vi "Next command.vi"(8 "error in (no error)":errorcluster, 11 "Channel in":refnum<class "Channel.lvclass">) -> (0 "error out":errorcluster, 3 "Channel out":refnum<class "Channel.lvclass">)   [LabVIEW 2018, in "Channel.lvclass"]
uses:
  Channel.lvclass
  Channel.lvclass/Channel.ctl
  State Machine/State Machine.lvclass/State Machine.ctl
  File interpreter/File interpreter.lvclass
  RxTx/RxTx.lvclass
  Interface/Interface.lvclass
  State Machine/State Machine.lvclass
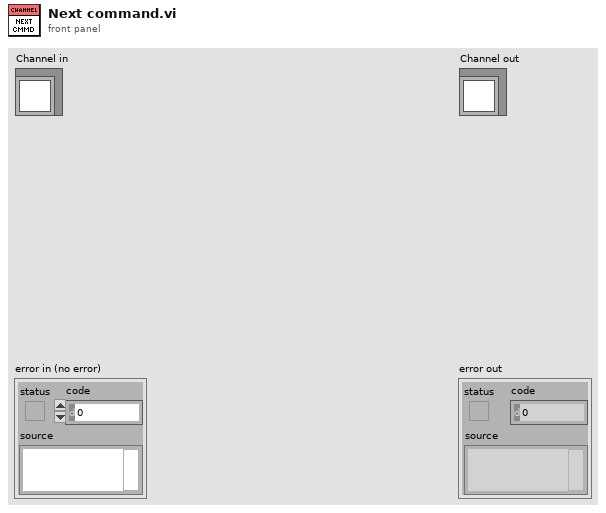
[diagram p1: front panel]
types:
  T1 = typedef "Shutter_mode typedef.ctl" = enum16{"Auto", "Open", "Close", "N/A (3)", "Open FVB Series", "Open Any Series"}
  T2 = typedef "ReadMode_mode typedef.ctl" = enum16{"Full Vertical Binning", "Multi-Track", "Random-Track", "Single-Track", "Image"}
  T3 = typedef "AcquisitionMode_mode typedef.ctl" = enum16{"Reserved (0)", "Single Scan", "Accumulate", "Kinetics", "Fast Kinetics", "Run Till Abort", "Reserved (6)", "Reserved (7)", "Reserved (8)", "Time Delayed Integration"}
  T4 = cluster{"EXPTIME":sgl, "PREAMP":enum16{"Gain 1", "Gain 2"}, "READOUT_RATE":enum16{"30 MHz", "20 MHz", "10 MHz", "1 MHz"}, "EM_GAIN":u16, "VBIN":u16, "INITIAL_LINE":u16, "INITIAL_COLUMN":u16, "FINAL_LINE":u16, "FINAL_COLUMN":u16, "#FRAMES":u32, "#CUBES":u32, "TRIGGER_MODE":enum16{"Internal", "External", "N/A", "N/A_1", "N/A_2", "N/A_3", "External Start"}, "HBIN":u16, "SHUTTER_TTL":enum16{"TTL Low", "TTL High"}, "SHUTTER_MODE":T1, "SHUTTER_OPENING_TIME":u16, "SHUTTER_CLOSING_TIME":u16, "VERTICAL_SHIFT_SPEED":u16, "READ_MODE":T2, "FRAME_TRANSFER":bool, "VERTICAL_CLOCK_VOLTAGE":enum16{"0", "+1", "+2", "+3", "+4"}, "ACQUISITION_MODE":T3, "AD_CHANNEL":u16, "EM_MODE":enum16{"Electron Multiplying", "Conventional"}}
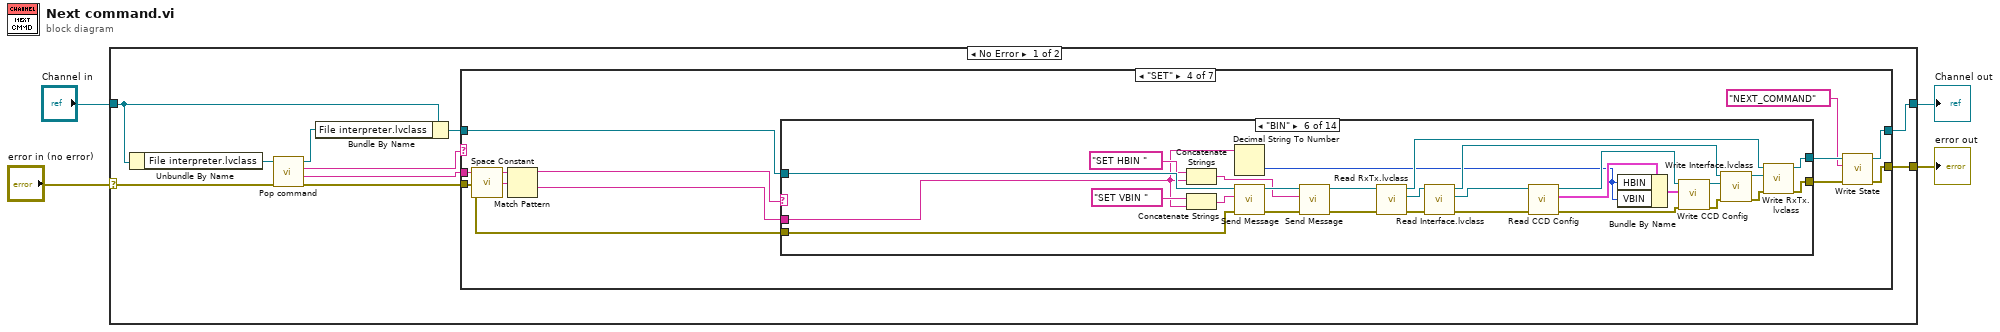
[diagram p0: block diagram]
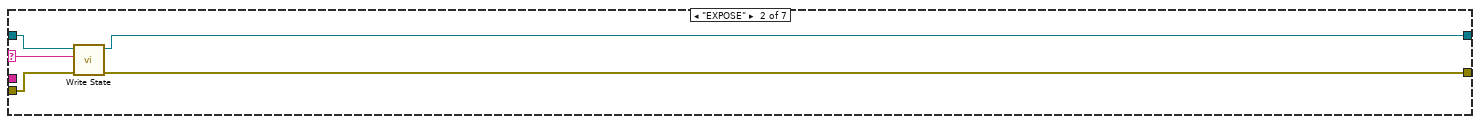
[diagram p3: hidden frame]
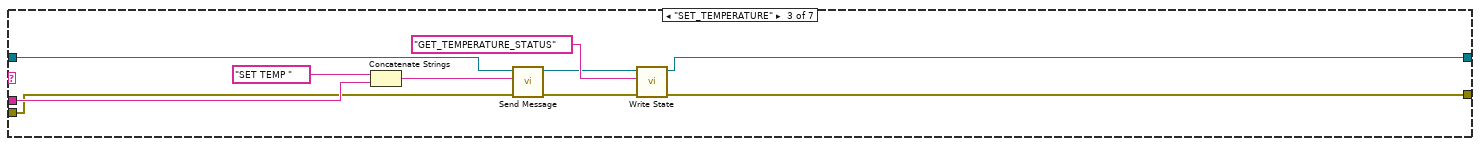
[diagram p4: hidden frame]
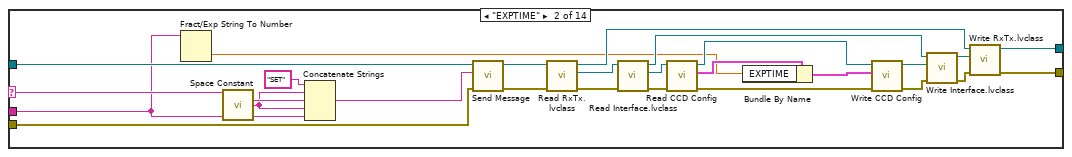
[diagram p6: hidden frame]
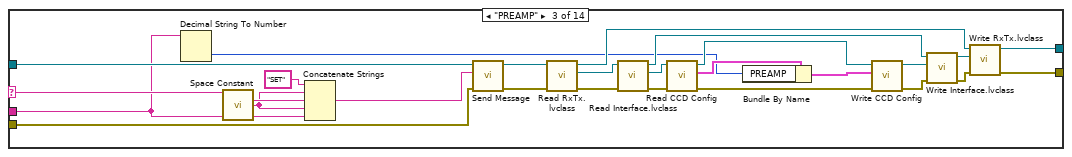
[diagram p7: hidden frame]
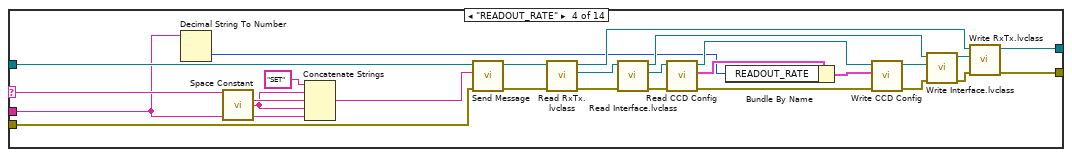
[diagram p8: hidden frame]
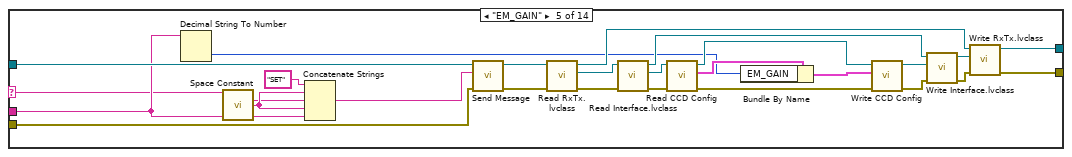
[diagram p9: hidden frame]
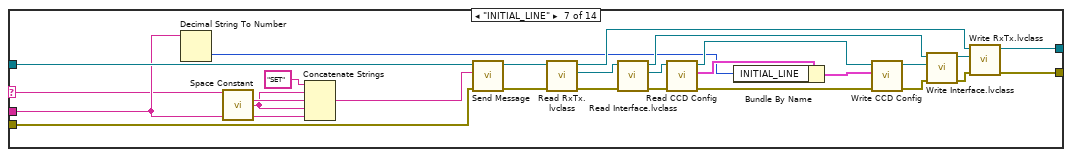
[diagram p10: hidden frame]
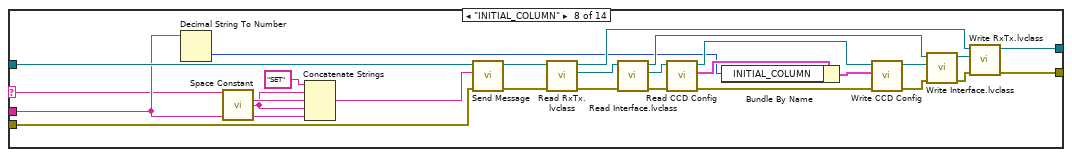
[diagram p11: hidden frame]
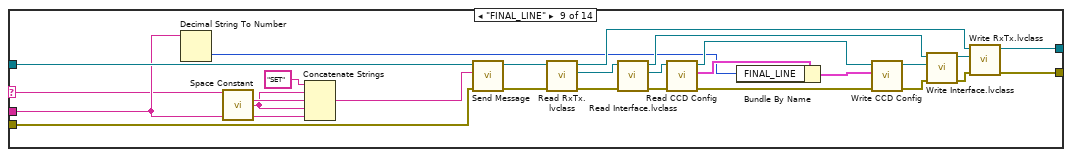
[diagram p12: hidden frame]
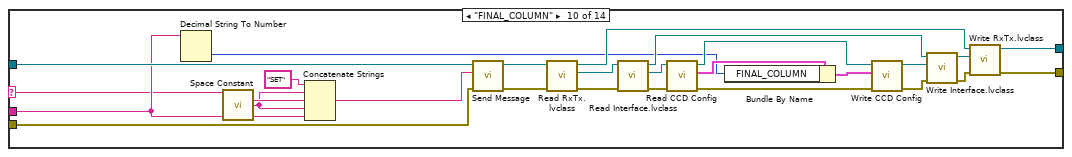
[diagram p13: hidden frame]
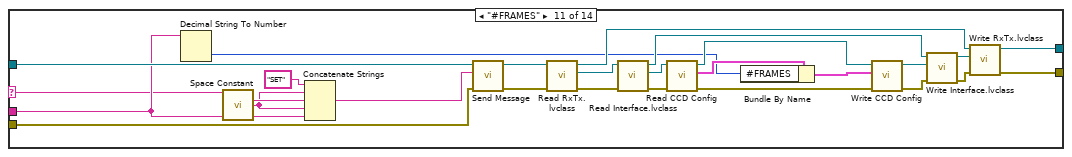
[diagram p14: hidden frame]
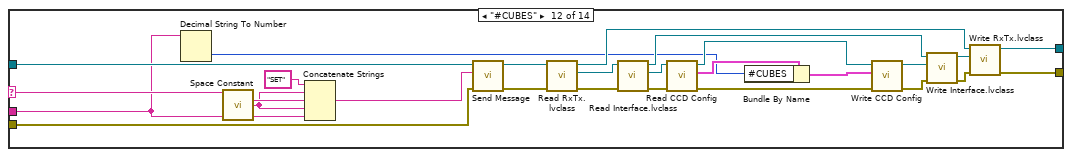
[diagram p15: hidden frame]
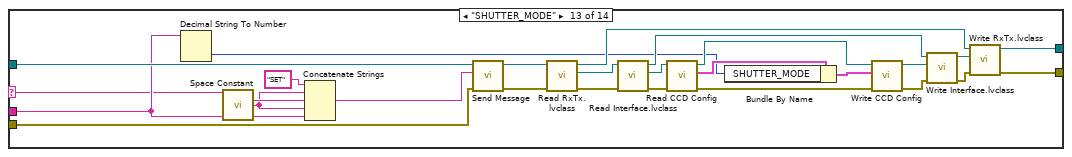
[diagram p16: hidden frame]
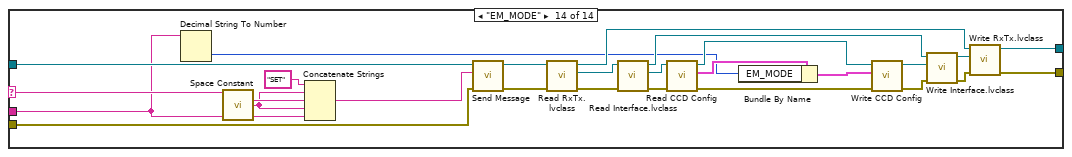
[diagram p17: hidden frame]
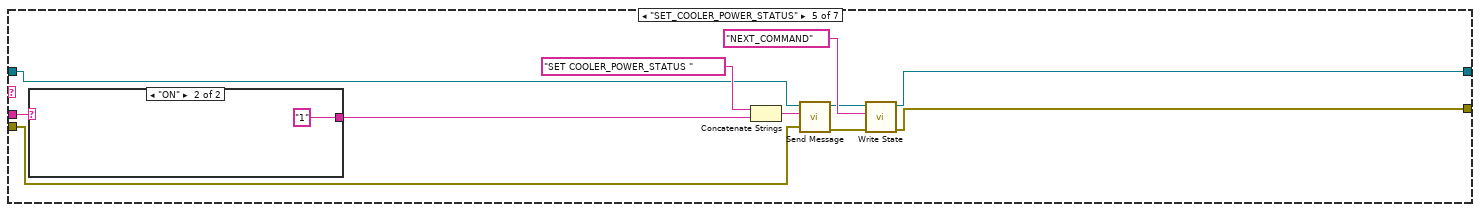
[diagram p18: hidden frame]
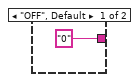
[diagram p19: hidden frame]
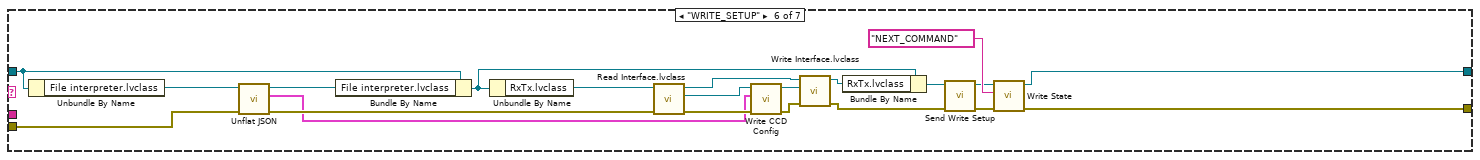
[diagram p20: hidden frame]
diagram:
  n1 = case shown="No Error" "error in (no error)" {
    selector: "error in (no error)" -> [w14 w433]
    tunnel: [w8 w433] -> w3
    tunnel: [w9 w432] -> w1
    tunnel: "Channel in" -> [w11 w432]
    frame No Error {
      n2 = Unbundle By Name(w11) -> ("File interpreter.lvclass"=w13:refnum<class "File interpreter.lvclass">)
      n3 = call "Pop command.vi"("error in (no error)"=w14, "File interpreter in"=w13) -> ("error out"=w10:errorcluster, "Value"=w5:string, "command"=w6:string, "File interpreter out"=w12:refnum<class "File interpreter.lvclass">)  [unwired: 6 in]
      n4 = Bundle By Name(cluster=w11, "File interpreter.lvclass"=w12) -> (w7:refnum<class "Channel.lvclass">)
      n5 = case shown="\"SET\"" w6 {
        selector: w6 -> [_ w17 _ _ _ _ _]
        tunnel: w7 -> [w16 w21 w25 w42 w390 w415 w431]
        tunnel: w10 -> [w15 w20 w22 w41 w387 w418 w428]
        tunnel: [w16 w19 w31 w35 w395 w403 w422] -> w9
        tunnel: [w15 w18 w30 w34 w394 w404 w421] -> w8
        tunnel: w5 -> [_ _ w26 w40 w386 _ w427]
        frame "False", Default {
        }
        frame "EXPOSE" {
          n6 = call "Write State.vi"("error in (no error)"=w20, "State"=w17, "Channel in"=w21) -> ("error out"=w18:errorcluster, "Channel out"=w19:refnum<class "Channel.lvclass">)  [unwired: 7 in]
        }
        frame "SET_TEMPERATURE" {
          n7 = Concatenate Strings("SET TEMP ", w26) -> (w28:string)
          n8 = call "Send Message.vi"("error in (no error)"=w22, "message"=w28, "Channel in"=w25) -> ("error out"=w23:errorcluster, "Channel out"=w24:refnum<class "Channel.lvclass">)  [unwired: 7 in]
          n9 = call "Write State.vi"("error in (no error)"=w23, "State"="GET_TEMPERATURE_STATUS", "Channel in"=w24) -> ("error out"=w30:errorcluster, "Channel out"=w31:refnum<class "Channel.lvclass">)  [unwired: 7 in]
        }
        frame "SET" {
          n10 = call <vilib>:"Space Constant.vi"() -> ("String"=w39:string)
          n11 = Match Pattern(string=w40, regular expression=w39) -> (before substring=w38:string, after substring=w37:string)  [unwired: 1 in, 2 out]
          n12 = case shown="\"BIN\"" w38 {
            selector: w38 -> [_ w48 w74 w100 w123 _ w179 w205 w231 w257 w283 w310 w335 w362]
            tunnel: [w44 w58 w84 w110 w136 w164 w190 w216 w242 w268 w294 w320 w346 w372] -> w36
            tunnel: [w43 w57 w83 w109 w135 w163 w189 w215 w241 w267 w293 w319 w345 w371] -> w33
            tunnel: w42 -> [w44 w51 w77 w103 w129 w160 w184 w210 w236 w262 w288 w314 w340 w366]
            tunnel: w41 -> [w43 w50 w76 w102 w128 w159 w183 w209 w235 w261 w287 w313 w339 w365]
            tunnel: w37 -> [_ w47 w73 w99 w126 w149 w180 w206 w232 w258 w284 w307 w336 w359]
            frame "False", Default {
            }
            frame "EXPTIME" {
              n13 = Fract/Exp String To Number(string=w47) -> (number=w54:dbl)  [unwired: 3 in, 1 out]
              n14 = call <vilib>:"Space Constant.vi"() -> ("String"=w46:string)
              n15 = Concatenate Strings("SET" ("string"), w46, w48, w46, w47) -> (w49:string)
              n16 = call "Send Message.vi"("error in (no error)"=w50, "message"=w49, "Channel in"=w51) -> ("error out"=w52:errorcluster, "Channel out"=w53:refnum<class "Channel.lvclass">)  [unwired: 7 in]
              n17 = call "Read RxTx.lvclass.vi"("error in (no error)"=w52, "Channel in"=w53) -> ("error out"=w60:errorcluster, "RxTx.lvclass"=w70:refnum<class "RxTx.lvclass">, "Channel out"=w65:refnum<class "Channel.lvclass">)  [unwired: 7 in]
              n18 = call "Read Interface.lvclass.vi"("error in (no error)"=w60, "RxTx in"=w70) -> ("error out"=w61:errorcluster, "Interface.lvclass"=w69:refnum<class "Interface.lvclass">, "RxTx out"=w64:refnum<class "RxTx.lvclass">)  [unwired: 7 in]
              n19 = call "Read CCD Config.vi"("error in (no error)"=w61, "Interface in"=w69) -> ("error out"=w59:errorcluster, "CCD Config"=w56:T4, "Interface out"=w68:refnum<class "Interface.lvclass">)  [unwired: 7 in]
              n20 = Bundle By Name(cluster=w56, "EXPTIME"=w54) -> (w55:T4)
              n21 = call "Write CCD Config.vi"("error in (no error)"=w59, "CCD Config"=w55, "Interface in"=w68) -> ("error out"=w62:errorcluster, "Interface out"=w67:refnum<class "Interface.lvclass">)  [unwired: 7 in]
              n22 = call "Write Interface.lvclass.vi"("error in (no error)"=w62, "Interface.lvclass"=w67, "RxTx in"=w64) -> ("error out"=w63:errorcluster, "RxTx out"=w66:refnum<class "RxTx.lvclass">)  [unwired: 7 in]
              n23 = call "Write RxTx.lvclass.vi"("error in (no error)"=w63, "RxTx.lvclass"=w66, "Channel in"=w65) -> ("error out"=w57:errorcluster, "Channel out"=w58:refnum<class "Channel.lvclass">)  [unwired: 7 in]
            }
            frame "PREAMP" {
              n24 = Decimal String To Number(string=w73) -> (number=w80:i32)  [unwired: 2 in, 1 out]
              n25 = call <vilib>:"Space Constant.vi"() -> ("String"=w72:string)
              n26 = Concatenate Strings("SET" ("string"), w72, w74, w72, w73) -> (w75:string)
              n27 = call "Send Message.vi"("error in (no error)"=w76, "message"=w75, "Channel in"=w77) -> ("error out"=w78:errorcluster, "Channel out"=w79:refnum<class "Channel.lvclass">)  [unwired: 7 in]
              n28 = call "Read RxTx.lvclass.vi"("error in (no error)"=w78, "Channel in"=w79) -> ("error out"=w86:errorcluster, "RxTx.lvclass"=w96:refnum<class "RxTx.lvclass">, "Channel out"=w91:refnum<class "Channel.lvclass">)  [unwired: 7 in]
              n29 = call "Read Interface.lvclass.vi"("error in (no error)"=w86, "RxTx in"=w96) -> ("error out"=w87:errorcluster, "Interface.lvclass"=w95:refnum<class "Interface.lvclass">, "RxTx out"=w90:refnum<class "RxTx.lvclass">)  [unwired: 7 in]
              n30 = call "Read CCD Config.vi"("error in (no error)"=w87, "Interface in"=w95) -> ("error out"=w85:errorcluster, "CCD Config"=w82:T4, "Interface out"=w94:refnum<class "Interface.lvclass">)  [unwired: 7 in]
              n31 = Bundle By Name(cluster=w82, "PREAMP"=w80) -> (w81:T4)
              n32 = call "Write CCD Config.vi"("error in (no error)"=w85, "CCD Config"=w81, "Interface in"=w94) -> ("error out"=w88:errorcluster, "Interface out"=w93:refnum<class "Interface.lvclass">)  [unwired: 7 in]
              n33 = call "Write Interface.lvclass.vi"("error in (no error)"=w88, "Interface.lvclass"=w93, "RxTx in"=w90) -> ("error out"=w89:errorcluster, "RxTx out"=w92:refnum<class "RxTx.lvclass">)  [unwired: 7 in]
              n34 = call "Write RxTx.lvclass.vi"("error in (no error)"=w89, "RxTx.lvclass"=w92, "Channel in"=w91) -> ("error out"=w83:errorcluster, "Channel out"=w84:refnum<class "Channel.lvclass">)  [unwired: 7 in]
            }
            frame "READOUT_RATE" {
              n35 = Decimal String To Number(string=w99) -> (number=w106:i32)  [unwired: 2 in, 1 out]
              n36 = call <vilib>:"Space Constant.vi"() -> ("String"=w98:string)
              n37 = Concatenate Strings("SET" ("string"), w98, w100, w98, w99) -> (w101:string)
              n38 = call "Send Message.vi"("error in (no error)"=w102, "message"=w101, "Channel in"=w103) -> ("error out"=w104:errorcluster, "Channel out"=w105:refnum<class "Channel.lvclass">)  [unwired: 7 in]
              n39 = call "Read RxTx.lvclass.vi"("error in (no error)"=w104, "Channel in"=w105) -> ("error out"=w112:errorcluster, "RxTx.lvclass"=w122:refnum<class "RxTx.lvclass">, "Channel out"=w117:refnum<class "Channel.lvclass">)  [unwired: 7 in]
              n40 = call "Read Interface.lvclass.vi"("error in (no error)"=w112, "RxTx in"=w122) -> ("error out"=w113:errorcluster, "Interface.lvclass"=w121:refnum<class "Interface.lvclass">, "RxTx out"=w116:refnum<class "RxTx.lvclass">)  [unwired: 7 in]
              n41 = call "Read CCD Config.vi"("error in (no error)"=w113, "Interface in"=w121) -> ("error out"=w111:errorcluster, "CCD Config"=w108:T4, "Interface out"=w120:refnum<class "Interface.lvclass">)  [unwired: 7 in]
              n42 = Bundle By Name(cluster=w108, "READOUT_RATE"=w106) -> (w107:T4)
              n43 = call "Write CCD Config.vi"("error in (no error)"=w111, "CCD Config"=w107, "Interface in"=w120) -> ("error out"=w114:errorcluster, "Interface out"=w119:refnum<class "Interface.lvclass">)  [unwired: 7 in]
              n44 = call "Write Interface.lvclass.vi"("error in (no error)"=w114, "Interface.lvclass"=w119, "RxTx in"=w116) -> ("error out"=w115:errorcluster, "RxTx out"=w118:refnum<class "RxTx.lvclass">)  [unwired: 7 in]
              n45 = call "Write RxTx.lvclass.vi"("error in (no error)"=w115, "RxTx.lvclass"=w118, "Channel in"=w117) -> ("error out"=w109:errorcluster, "Channel out"=w110:refnum<class "Channel.lvclass">)  [unwired: 7 in]
            }
            frame "EM_GAIN" {
              n46 = Decimal String To Number(string=w126) -> (number=w132:i32)  [unwired: 2 in, 1 out]
              n47 = call <vilib>:"Space Constant.vi"() -> ("String"=w124:string)
              n48 = Concatenate Strings("SET" ("string"), w124, w123, w124, w126) -> (w127:string)
              n49 = call "Send Message.vi"("error in (no error)"=w128, "message"=w127, "Channel in"=w129) -> ("error out"=w130:errorcluster, "Channel out"=w131:refnum<class "Channel.lvclass">)  [unwired: 7 in]
              n50 = call "Read RxTx.lvclass.vi"("error in (no error)"=w130, "Channel in"=w131) -> ("error out"=w138:errorcluster, "RxTx.lvclass"=w148:refnum<class "RxTx.lvclass">, "Channel out"=w143:refnum<class "Channel.lvclass">)  [unwired: 7 in]
              n51 = call "Read Interface.lvclass.vi"("error in (no error)"=w138, "RxTx in"=w148) -> ("error out"=w139:errorcluster, "Interface.lvclass"=w147:refnum<class "Interface.lvclass">, "RxTx out"=w142:refnum<class "RxTx.lvclass">)  [unwired: 7 in]
              n52 = call "Read CCD Config.vi"("error in (no error)"=w139, "Interface in"=w147) -> ("error out"=w137:errorcluster, "CCD Config"=w134:T4, "Interface out"=w146:refnum<class "Interface.lvclass">)  [unwired: 7 in]
              n53 = Bundle By Name(cluster=w134, "EM_GAIN"=w132) -> (w133:T4)
              n54 = call "Write CCD Config.vi"("error in (no error)"=w137, "CCD Config"=w133, "Interface in"=w146) -> ("error out"=w140:errorcluster, "Interface out"=w145:refnum<class "Interface.lvclass">)  [unwired: 7 in]
              n55 = call "Write Interface.lvclass.vi"("error in (no error)"=w140, "Interface.lvclass"=w145, "RxTx in"=w142) -> ("error out"=w141:errorcluster, "RxTx out"=w144:refnum<class "RxTx.lvclass">)  [unwired: 7 in]
              n56 = call "Write RxTx.lvclass.vi"("error in (no error)"=w141, "RxTx.lvclass"=w144, "Channel in"=w143) -> ("error out"=w135:errorcluster, "Channel out"=w136:refnum<class "Channel.lvclass">)  [unwired: 7 in]
            }
            frame "BIN" {
              n57 = Concatenate Strings("SET HBIN " ("string"), w149) -> (w150:string)
              n58 = Concatenate Strings("SET VBIN " ("string"), w149) -> (w158:string)
              n59 = Decimal String To Number(string=w149) -> (number=w157:i32)  [unwired: 2 in, 1 out]
              n60 = call "Send Message.vi"("error in (no error)"=w159, "message"=w158, "Channel in"=w160) -> ("error out"=w152:errorcluster, "Channel out"=w155:refnum<class "Channel.lvclass">)  [unwired: 7 in]
              n61 = call "Send Message.vi"("error in (no error)"=w152, "message"=w150, "Channel in"=w155) -> ("error out"=w153:errorcluster, "Channel out"=w154:refnum<class "Channel.lvclass">)  [unwired: 7 in]
              n62 = call "Read RxTx.lvclass.vi"("error in (no error)"=w153, "Channel in"=w154) -> ("error out"=w166:errorcluster, "RxTx.lvclass"=w176:refnum<class "RxTx.lvclass">, "Channel out"=w171:refnum<class "Channel.lvclass">)  [unwired: 7 in]
              n63 = call "Read Interface.lvclass.vi"("error in (no error)"=w166, "RxTx in"=w176) -> ("error out"=w167:errorcluster, "Interface.lvclass"=w175:refnum<class "Interface.lvclass">, "RxTx out"=w170:refnum<class "RxTx.lvclass">)  [unwired: 7 in]
              n64 = call "Read CCD Config.vi"("error in (no error)"=w167, "Interface in"=w175) -> ("error out"=w165:errorcluster, "CCD Config"=w162:T4, "Interface out"=w174:refnum<class "Interface.lvclass">)  [unwired: 7 in]
              n65 = Bundle By Name(cluster=w162, "HBIN"=w157, "VBIN"=w157) -> (w161:T4)
              n66 = call "Write CCD Config.vi"("error in (no error)"=w165, "CCD Config"=w161, "Interface in"=w174) -> ("error out"=w168:errorcluster, "Interface out"=w173:refnum<class "Interface.lvclass">)  [unwired: 7 in]
              n67 = call "Write Interface.lvclass.vi"("error in (no error)"=w168, "Interface.lvclass"=w173, "RxTx in"=w170) -> ("error out"=w169:errorcluster, "RxTx out"=w172:refnum<class "RxTx.lvclass">)  [unwired: 7 in]
              n68 = call "Write RxTx.lvclass.vi"("error in (no error)"=w169, "RxTx.lvclass"=w172, "Channel in"=w171) -> ("error out"=w163:errorcluster, "Channel out"=w164:refnum<class "Channel.lvclass">)  [unwired: 7 in]
            }
            frame "INITIAL_LINE" {
              n69 = Decimal String To Number(string=w180) -> (number=w181:i32)  [unwired: 2 in, 1 out]
              n70 = call <vilib>:"Space Constant.vi"() -> ("String"=w178:string)
              n71 = Concatenate Strings("SET" ("string"), w178, w179, w178, w180) -> (w182:string)
              n72 = call "Send Message.vi"("error in (no error)"=w183, "message"=w182, "Channel in"=w184) -> ("error out"=w185:errorcluster, "Channel out"=w186:refnum<class "Channel.lvclass">)  [unwired: 7 in]
              n73 = call "Read RxTx.lvclass.vi"("error in (no error)"=w185, "Channel in"=w186) -> ("error out"=w192:errorcluster, "RxTx.lvclass"=w202:refnum<class "RxTx.lvclass">, "Channel out"=w197:refnum<class "Channel.lvclass">)  [unwired: 7 in]
              n74 = call "Read Interface.lvclass.vi"("error in (no error)"=w192, "RxTx in"=w202) -> ("error out"=w193:errorcluster, "Interface.lvclass"=w201:refnum<class "Interface.lvclass">, "RxTx out"=w196:refnum<class "RxTx.lvclass">)  [unwired: 7 in]
              n75 = call "Read CCD Config.vi"("error in (no error)"=w193, "Interface in"=w201) -> ("error out"=w191:errorcluster, "CCD Config"=w188:T4, "Interface out"=w200:refnum<class "Interface.lvclass">)  [unwired: 7 in]
              n76 = Bundle By Name(cluster=w188, "INITIAL_LINE"=w181) -> (w187:T4)
              n77 = call "Write CCD Config.vi"("error in (no error)"=w191, "CCD Config"=w187, "Interface in"=w200) -> ("error out"=w194:errorcluster, "Interface out"=w199:refnum<class "Interface.lvclass">)  [unwired: 7 in]
              n78 = call "Write Interface.lvclass.vi"("error in (no error)"=w194, "Interface.lvclass"=w199, "RxTx in"=w196) -> ("error out"=w195:errorcluster, "RxTx out"=w198:refnum<class "RxTx.lvclass">)  [unwired: 7 in]
              n79 = call "Write RxTx.lvclass.vi"("error in (no error)"=w195, "RxTx.lvclass"=w198, "Channel in"=w197) -> ("error out"=w189:errorcluster, "Channel out"=w190:refnum<class "Channel.lvclass">)  [unwired: 7 in]
            }
            frame "INITIAL_COLUMN" {
              n80 = Decimal String To Number(string=w206) -> (number=w207:i32)  [unwired: 2 in, 1 out]
              n81 = call <vilib>:"Space Constant.vi"() -> ("String"=w204:string)
              n82 = Concatenate Strings("SET" ("string"), w204, w205, w204, w206) -> (w208:string)
              n83 = call "Send Message.vi"("error in (no error)"=w209, "message"=w208, "Channel in"=w210) -> ("error out"=w211:errorcluster, "Channel out"=w212:refnum<class "Channel.lvclass">)  [unwired: 7 in]
              n84 = call "Read RxTx.lvclass.vi"("error in (no error)"=w211, "Channel in"=w212) -> ("error out"=w218:errorcluster, "RxTx.lvclass"=w228:refnum<class "RxTx.lvclass">, "Channel out"=w223:refnum<class "Channel.lvclass">)  [unwired: 7 in]
              n85 = call "Read Interface.lvclass.vi"("error in (no error)"=w218, "RxTx in"=w228) -> ("error out"=w219:errorcluster, "Interface.lvclass"=w227:refnum<class "Interface.lvclass">, "RxTx out"=w222:refnum<class "RxTx.lvclass">)  [unwired: 7 in]
              n86 = call "Read CCD Config.vi"("error in (no error)"=w219, "Interface in"=w227) -> ("error out"=w217:errorcluster, "CCD Config"=w214:T4, "Interface out"=w226:refnum<class "Interface.lvclass">)  [unwired: 7 in]
              n87 = Bundle By Name(cluster=w214, "INITIAL_COLUMN"=w207) -> (w213:T4)
              n88 = call "Write CCD Config.vi"("error in (no error)"=w217, "CCD Config"=w213, "Interface in"=w226) -> ("error out"=w220:errorcluster, "Interface out"=w225:refnum<class "Interface.lvclass">)  [unwired: 7 in]
              n89 = call "Write Interface.lvclass.vi"("error in (no error)"=w220, "Interface.lvclass"=w225, "RxTx in"=w222) -> ("error out"=w221:errorcluster, "RxTx out"=w224:refnum<class "RxTx.lvclass">)  [unwired: 7 in]
              n90 = call "Write RxTx.lvclass.vi"("error in (no error)"=w221, "RxTx.lvclass"=w224, "Channel in"=w223) -> ("error out"=w215:errorcluster, "Channel out"=w216:refnum<class "Channel.lvclass">)  [unwired: 7 in]
            }
            frame "FINAL_LINE" {
              n91 = Decimal String To Number(string=w232) -> (number=w233:i32)  [unwired: 2 in, 1 out]
              n92 = call <vilib>:"Space Constant.vi"() -> ("String"=w230:string)
              n93 = Concatenate Strings("SET" ("string"), w230, w231, w230, w232) -> (w234:string)
              n94 = call "Send Message.vi"("error in (no error)"=w235, "message"=w234, "Channel in"=w236) -> ("error out"=w237:errorcluster, "Channel out"=w238:refnum<class "Channel.lvclass">)  [unwired: 7 in]
              n95 = call "Read RxTx.lvclass.vi"("error in (no error)"=w237, "Channel in"=w238) -> ("error out"=w244:errorcluster, "RxTx.lvclass"=w254:refnum<class "RxTx.lvclass">, "Channel out"=w249:refnum<class "Channel.lvclass">)  [unwired: 7 in]
              n96 = call "Read Interface.lvclass.vi"("error in (no error)"=w244, "RxTx in"=w254) -> ("error out"=w245:errorcluster, "Interface.lvclass"=w253:refnum<class "Interface.lvclass">, "RxTx out"=w248:refnum<class "RxTx.lvclass">)  [unwired: 7 in]
              n97 = call "Read CCD Config.vi"("error in (no error)"=w245, "Interface in"=w253) -> ("error out"=w243:errorcluster, "CCD Config"=w240:T4, "Interface out"=w252:refnum<class "Interface.lvclass">)  [unwired: 7 in]
              n98 = Bundle By Name(cluster=w240, "FINAL_LINE"=w233) -> (w239:T4)
              n99 = call "Write CCD Config.vi"("error in (no error)"=w243, "CCD Config"=w239, "Interface in"=w252) -> ("error out"=w246:errorcluster, "Interface out"=w251:refnum<class "Interface.lvclass">)  [unwired: 7 in]
              n100 = call "Write Interface.lvclass.vi"("error in (no error)"=w246, "Interface.lvclass"=w251, "RxTx in"=w248) -> ("error out"=w247:errorcluster, "RxTx out"=w250:refnum<class "RxTx.lvclass">)  [unwired: 7 in]
              n101 = call "Write RxTx.lvclass.vi"("error in (no error)"=w247, "RxTx.lvclass"=w250, "Channel in"=w249) -> ("error out"=w241:errorcluster, "Channel out"=w242:refnum<class "Channel.lvclass">)  [unwired: 7 in]
            }
            frame "FINAL_COLUMN" {
              n102 = Decimal String To Number(string=w258) -> (number=w259:i32)  [unwired: 2 in, 1 out]
              n103 = call <vilib>:"Space Constant.vi"() -> ("String"=w256:string)
              n104 = Concatenate Strings("SET" ("string"), w256, w257, w256, w258) -> (w260:string)
              n105 = call "Send Message.vi"("error in (no error)"=w261, "message"=w260, "Channel in"=w262) -> ("error out"=w263:errorcluster, "Channel out"=w264:refnum<class "Channel.lvclass">)  [unwired: 7 in]
              n106 = call "Read RxTx.lvclass.vi"("error in (no error)"=w263, "Channel in"=w264) -> ("error out"=w270:errorcluster, "RxTx.lvclass"=w280:refnum<class "RxTx.lvclass">, "Channel out"=w275:refnum<class "Channel.lvclass">)  [unwired: 7 in]
              n107 = call "Read Interface.lvclass.vi"("error in (no error)"=w270, "RxTx in"=w280) -> ("error out"=w271:errorcluster, "Interface.lvclass"=w279:refnum<class "Interface.lvclass">, "RxTx out"=w274:refnum<class "RxTx.lvclass">)  [unwired: 7 in]
              n108 = call "Read CCD Config.vi"("error in (no error)"=w271, "Interface in"=w279) -> ("error out"=w269:errorcluster, "CCD Config"=w266:T4, "Interface out"=w278:refnum<class "Interface.lvclass">)  [unwired: 7 in]
              n109 = Bundle By Name(cluster=w266, "FINAL_COLUMN"=w259) -> (w265:T4)
              n110 = call "Write CCD Config.vi"("error in (no error)"=w269, "CCD Config"=w265, "Interface in"=w278) -> ("error out"=w272:errorcluster, "Interface out"=w277:refnum<class "Interface.lvclass">)  [unwired: 7 in]
              n111 = call "Write Interface.lvclass.vi"("error in (no error)"=w272, "Interface.lvclass"=w277, "RxTx in"=w274) -> ("error out"=w273:errorcluster, "RxTx out"=w276:refnum<class "RxTx.lvclass">)  [unwired: 7 in]
              n112 = call "Write RxTx.lvclass.vi"("error in (no error)"=w273, "RxTx.lvclass"=w276, "Channel in"=w275) -> ("error out"=w267:errorcluster, "Channel out"=w268:refnum<class "Channel.lvclass">)  [unwired: 7 in]
            }
            frame "#FRAMES" {
              n113 = Decimal String To Number(string=w284) -> (number=w285:i32)  [unwired: 2 in, 1 out]
              n114 = call <vilib>:"Space Constant.vi"() -> ("String"=w282:string)
              n115 = Concatenate Strings("SET" ("string"), w282, w283, w282, w284) -> (w286:string)
              n116 = call "Send Message.vi"("error in (no error)"=w287, "message"=w286, "Channel in"=w288) -> ("error out"=w289:errorcluster, "Channel out"=w290:refnum<class "Channel.lvclass">)  [unwired: 7 in]
              n117 = call "Read RxTx.lvclass.vi"("error in (no error)"=w289, "Channel in"=w290) -> ("error out"=w296:errorcluster, "RxTx.lvclass"=w306:refnum<class "RxTx.lvclass">, "Channel out"=w301:refnum<class "Channel.lvclass">)  [unwired: 7 in]
              n118 = call "Read Interface.lvclass.vi"("error in (no error)"=w296, "RxTx in"=w306) -> ("error out"=w297:errorcluster, "Interface.lvclass"=w305:refnum<class "Interface.lvclass">, "RxTx out"=w300:refnum<class "RxTx.lvclass">)  [unwired: 7 in]
              n119 = call "Read CCD Config.vi"("error in (no error)"=w297, "Interface in"=w305) -> ("error out"=w295:errorcluster, "CCD Config"=w292:T4, "Interface out"=w304:refnum<class "Interface.lvclass">)  [unwired: 7 in]
              n120 = Bundle By Name(cluster=w292, "#FRAMES"=w285) -> (w291:T4)
              n121 = call "Write CCD Config.vi"("error in (no error)"=w295, "CCD Config"=w291, "Interface in"=w304) -> ("error out"=w298:errorcluster, "Interface out"=w303:refnum<class "Interface.lvclass">)  [unwired: 7 in]
              n122 = call "Write Interface.lvclass.vi"("error in (no error)"=w298, "Interface.lvclass"=w303, "RxTx in"=w300) -> ("error out"=w299:errorcluster, "RxTx out"=w302:refnum<class "RxTx.lvclass">)  [unwired: 7 in]
              n123 = call "Write RxTx.lvclass.vi"("error in (no error)"=w299, "RxTx.lvclass"=w302, "Channel in"=w301) -> ("error out"=w293:errorcluster, "Channel out"=w294:refnum<class "Channel.lvclass">)  [unwired: 7 in]
            }
            frame "#CUBES" {
              n124 = Decimal String To Number(string=w307) -> (number=w311:i32)  [unwired: 2 in, 1 out]
              n125 = call <vilib>:"Space Constant.vi"() -> ("String"=w309:string)
              n126 = Concatenate Strings("SET" ("string"), w309, w310, w309, w307) -> (w312:string)
              n127 = call "Send Message.vi"("error in (no error)"=w313, "message"=w312, "Channel in"=w314) -> ("error out"=w315:errorcluster, "Channel out"=w316:refnum<class "Channel.lvclass">)  [unwired: 7 in]
              n128 = call "Read RxTx.lvclass.vi"("error in (no error)"=w315, "Channel in"=w316) -> ("error out"=w322:errorcluster, "RxTx.lvclass"=w332:refnum<class "RxTx.lvclass">, "Channel out"=w327:refnum<class "Channel.lvclass">)  [unwired: 7 in]
              n129 = call "Read Interface.lvclass.vi"("error in (no error)"=w322, "RxTx in"=w332) -> ("error out"=w323:errorcluster, "Interface.lvclass"=w331:refnum<class "Interface.lvclass">, "RxTx out"=w326:refnum<class "RxTx.lvclass">)  [unwired: 7 in]
              n130 = call "Read CCD Config.vi"("error in (no error)"=w323, "Interface in"=w331) -> ("error out"=w321:errorcluster, "CCD Config"=w318:T4, "Interface out"=w330:refnum<class "Interface.lvclass">)  [unwired: 7 in]
              n131 = Bundle By Name(cluster=w318, "#CUBES"=w311) -> (w317:T4)
              n132 = call "Write CCD Config.vi"("error in (no error)"=w321, "CCD Config"=w317, "Interface in"=w330) -> ("error out"=w324:errorcluster, "Interface out"=w329:refnum<class "Interface.lvclass">)  [unwired: 7 in]
              n133 = call "Write Interface.lvclass.vi"("error in (no error)"=w324, "Interface.lvclass"=w329, "RxTx in"=w326) -> ("error out"=w325:errorcluster, "RxTx out"=w328:refnum<class "RxTx.lvclass">)  [unwired: 7 in]
              n134 = call "Write RxTx.lvclass.vi"("error in (no error)"=w325, "RxTx.lvclass"=w328, "Channel in"=w327) -> ("error out"=w319:errorcluster, "Channel out"=w320:refnum<class "Channel.lvclass">)  [unwired: 7 in]
            }
            frame "SHUTTER_MODE" {
              n135 = Decimal String To Number(string=w336) -> (number=w337:i32)  [unwired: 2 in, 1 out]
              n136 = call <vilib>:"Space Constant.vi"() -> ("String"=w334:string)
              n137 = Concatenate Strings("SET" ("string"), w334, w335, w334, w336) -> (w338:string)
              n138 = call "Send Message.vi"("error in (no error)"=w339, "message"=w338, "Channel in"=w340) -> ("error out"=w341:errorcluster, "Channel out"=w342:refnum<class "Channel.lvclass">)  [unwired: 7 in]
              n139 = call "Read RxTx.lvclass.vi"("error in (no error)"=w341, "Channel in"=w342) -> ("error out"=w348:errorcluster, "RxTx.lvclass"=w358:refnum<class "RxTx.lvclass">, "Channel out"=w353:refnum<class "Channel.lvclass">)  [unwired: 7 in]
              n140 = call "Read Interface.lvclass.vi"("error in (no error)"=w348, "RxTx in"=w358) -> ("error out"=w349:errorcluster, "Interface.lvclass"=w357:refnum<class "Interface.lvclass">, "RxTx out"=w352:refnum<class "RxTx.lvclass">)  [unwired: 7 in]
              n141 = call "Read CCD Config.vi"("error in (no error)"=w349, "Interface in"=w357) -> ("error out"=w347:errorcluster, "CCD Config"=w344:T4, "Interface out"=w356:refnum<class "Interface.lvclass">)  [unwired: 7 in]
              n142 = Bundle By Name(cluster=w344, "SHUTTER_MODE"=w337) -> (w343:T4)
              n143 = call "Write CCD Config.vi"("error in (no error)"=w347, "CCD Config"=w343, "Interface in"=w356) -> ("error out"=w350:errorcluster, "Interface out"=w355:refnum<class "Interface.lvclass">)  [unwired: 7 in]
              n144 = call "Write Interface.lvclass.vi"("error in (no error)"=w350, "Interface.lvclass"=w355, "RxTx in"=w352) -> ("error out"=w351:errorcluster, "RxTx out"=w354:refnum<class "RxTx.lvclass">)  [unwired: 7 in]
              n145 = call "Write RxTx.lvclass.vi"("error in (no error)"=w351, "RxTx.lvclass"=w354, "Channel in"=w353) -> ("error out"=w345:errorcluster, "Channel out"=w346:refnum<class "Channel.lvclass">)  [unwired: 7 in]
            }
            frame "EM_MODE" {
              n146 = Decimal String To Number(string=w359) -> (number=w363:i32)  [unwired: 2 in, 1 out]
              n147 = call <vilib>:"Space Constant.vi"() -> ("String"=w361:string)
              n148 = Concatenate Strings("SET" ("string"), w361, w362, w361, w359) -> (w364:string)
              n149 = call "Send Message.vi"("error in (no error)"=w365, "message"=w364, "Channel in"=w366) -> ("error out"=w367:errorcluster, "Channel out"=w368:refnum<class "Channel.lvclass">)  [unwired: 7 in]
              n150 = call "Read RxTx.lvclass.vi"("error in (no error)"=w367, "Channel in"=w368) -> ("error out"=w374:errorcluster, "RxTx.lvclass"=w384:refnum<class "RxTx.lvclass">, "Channel out"=w379:refnum<class "Channel.lvclass">)  [unwired: 7 in]
              n151 = call "Read Interface.lvclass.vi"("error in (no error)"=w374, "RxTx in"=w384) -> ("error out"=w375:errorcluster, "Interface.lvclass"=w383:refnum<class "Interface.lvclass">, "RxTx out"=w378:refnum<class "RxTx.lvclass">)  [unwired: 7 in]
              n152 = call "Read CCD Config.vi"("error in (no error)"=w375, "Interface in"=w383) -> ("error out"=w373:errorcluster, "CCD Config"=w370:T4, "Interface out"=w382:refnum<class "Interface.lvclass">)  [unwired: 7 in]
              n153 = Bundle By Name(cluster=w370, "EM_MODE"=w363) -> (w369:T4)
              n154 = call "Write CCD Config.vi"("error in (no error)"=w373, "CCD Config"=w369, "Interface in"=w382) -> ("error out"=w376:errorcluster, "Interface out"=w381:refnum<class "Interface.lvclass">)  [unwired: 7 in]
              n155 = call "Write Interface.lvclass.vi"("error in (no error)"=w376, "Interface.lvclass"=w381, "RxTx in"=w378) -> ("error out"=w377:errorcluster, "RxTx out"=w380:refnum<class "RxTx.lvclass">)  [unwired: 7 in]
              n156 = call "Write RxTx.lvclass.vi"("error in (no error)"=w377, "RxTx.lvclass"=w380, "Channel in"=w379) -> ("error out"=w371:errorcluster, "Channel out"=w372:refnum<class "Channel.lvclass">)  [unwired: 7 in]
            }
          }
          n157 = call "Write State.vi"("error in (no error)"=w33, "State"="NEXT_COMMAND", "Channel in"=w36) -> ("error out"=w34:errorcluster, "Channel out"=w35:refnum<class "Channel.lvclass">)  [unwired: 7 in]
        }
        frame "SET_COOLER_POWER_STATUS" {
          n158 = case shown="\"ON\"" w386 {
            tunnel: ["0" "1"] -> w385
            frame "OFF", Default {
            }
            frame "ON" {
            }
          }
          n159 = Concatenate Strings("SET COOLER_POWER_STATUS ", w385) -> (w392:string)
          n160 = call "Send Message.vi"("error in (no error)"=w387, "message"=w392, "Channel in"=w390) -> ("error out"=w388:errorcluster, "Channel out"=w389:refnum<class "Channel.lvclass">)  [unwired: 7 in]
          n161 = call "Write State.vi"("error in (no error)"=w388, "State"="NEXT_COMMAND", "Channel in"=w389) -> ("error out"=w394:errorcluster, "Channel out"=w395:refnum<class "Channel.lvclass">)  [unwired: 7 in]
        }
        frame "WRITE_SETUP" {
          n162 = Unbundle By Name(w415) -> ("File interpreter.lvclass"=w417:refnum<class "File interpreter.lvclass">)
          n163 = call "Unflat JSON.vi"("error in (no error)"=w418, "File interpreter in"=w417) -> ("error out"=w413:errorcluster, "CCD Config"=w407:T4, "File interpreter out"=w416:refnum<class "File interpreter.lvclass">)  [unwired: 7 in]
          n164 = Bundle By Name(cluster=w415, "File interpreter.lvclass"=w416) -> (w406:refnum<class "Channel.lvclass">)
          n165 = Unbundle By Name(w406) -> ("RxTx.lvclass"=w414:refnum<class "RxTx.lvclass">)
          n166 = call "Read Interface.lvclass.vi"("error in (no error)"=w413, "RxTx in"=w414) -> ("error out"=w410:errorcluster, "Interface.lvclass"=w411:refnum<class "Interface.lvclass">, "RxTx out"=w408:refnum<class "RxTx.lvclass">)  [unwired: 7 in]
          n167 = call "Write CCD Config.vi"("error in (no error)"=w410, "CCD Config"=w407, "Interface in"=w411) -> ("error out"=w409:errorcluster, "Interface out"=w412:refnum<class "Interface.lvclass">)  [unwired: 7 in]
          n168 = call "Write Interface.lvclass.vi"("error in (no error)"=w409, "Interface.lvclass"=w412, "RxTx in"=w408) -> ("error out"=w398:errorcluster, "RxTx out"=w405:refnum<class "RxTx.lvclass">)  [unwired: 7 in]
          n169 = Bundle By Name(cluster=w406, "RxTx.lvclass"=w405) -> (w401:refnum<class "Channel.lvclass">)
          n170 = call "Send Write Setup.vi"("error in (no error)"=w398, "Channel in"=w401) -> ("error out"=w399:errorcluster, "Channel out"=w400:refnum<class "Channel.lvclass">)  [unwired: 8 in]
          n171 = call "Write State.vi"("error in (no error)"=w399, "State"="NEXT_COMMAND", "Channel in"=w400) -> ("error out"=w404:errorcluster, "Channel out"=w403:refnum<class "Channel.lvclass">)  [unwired: 7 in]
        }
        frame "SET_WAIT_TIME" {
          n172 = Decimal String To Number(string=w427) -> (number=w426:i32)  [unwired: 2 in, 1 out]
          n173 = Unbundle By Name(w431) -> ("State Machine.lvclass"=w430:refnum<class "State Machine.lvclass">)
          n174 = Multiply(x=1000, y=w426) -> (x*y=w425:i32)
          n175 = call "Write Limit Timer.vi"("error in (no error)"=w428, "Limit Timer"=w425, "State Machine in"=w430) -> ("error out"=w420:errorcluster, "State Machine out"=w429:refnum<class "State Machine.lvclass">)  [unwired: 7 in]
          n176 = Bundle By Name(cluster=w431, "State Machine.lvclass"=w429) -> (w423:refnum<class "Channel.lvclass">)
          n177 = call "Write State.vi"("error in (no error)"=w420, "State"="NEXT_COMMAND", "Channel in"=w423) -> ("error out"=w421:errorcluster, "Channel out"=w422:refnum<class "Channel.lvclass">)  [unwired: 7 in]
        }
      }
    }
    frame Error {
    }
  }
  "error out" <- w3
  "Channel out" <- w1
